vi "st_Poisson CDF (kx).vi"(10 "a":dbl=1.0, 11 "x":dbl=1.0) -> (0 "error":i32, 3 "cdf(x)":dbl=0.7357588823428847)   [LabVIEW 2020, in "NI_Gmath.lvlib"]
uses:
  <vilib>/gmath/NI_Gmath.lvlib
  <vilib>/gmath/statdist.llb/st_error_code.ctl
panel:
  # "Poisson CDF"
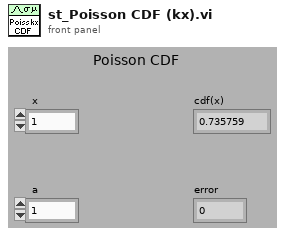
[diagram p1: front panel]
types:
  T1 = typedef "NI_Gmath.lvlib/st_error_code.ctl" = i32
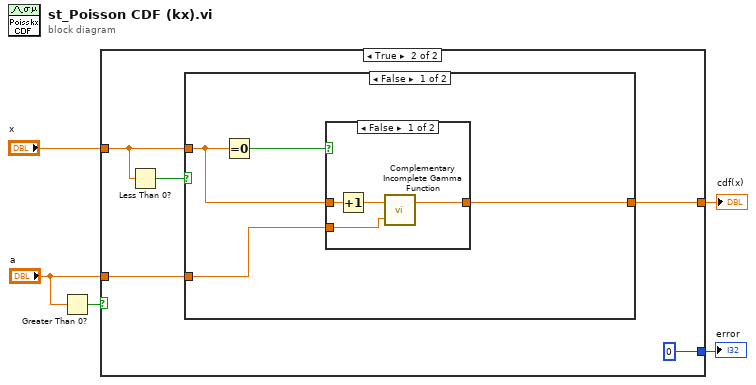
[diagram p0: block diagram]
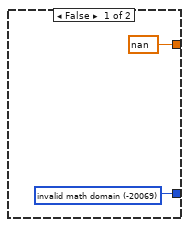
[diagram p2: hidden frame]
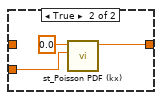
[diagram p3: hidden frame]
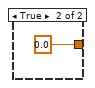
[diagram p4: hidden frame]
diagram:
  n1 = Greater Than 0?(x="a") -> (x > 0?=w1:bool)
  n2 = case shown="True" w1 {
    tunnel: [w6 0 ("invalid math domain")] -> w5
    tunnel: [nan w8] -> w4
    tunnel: "x" -> [_ w9]
    tunnel: "a" -> [_ w10]
    frame False {
      w6 = T1 -20069 items=["invalid math domain"=-20069, "Fourier interpolation size m >= n"=-20070, "empty array"=-20003] ("stat interp error code")
    }
    frame True {
      n3 = Less Than 0?(x=w9) -> (x < 0?=w11:bool)
      n4 = case shown="False" w11 {
        tunnel: [w13 0.0] -> w8
        tunnel: w10 -> [w14 _]
        tunnel: w9 -> [w16 _]
        frame False {
          n5 = Equal To 0?(x=w16) -> (x = 0?=w15:bool)
          n6 = case shown="False" w15 {
            tunnel: w16 -> [w20 _]
            tunnel: [w18 w21] -> w13
            tunnel: w14 -> [w17 w22]
            frame False {
              n7 = Increment(x=w20) -> (x+1=w19:dbl)
              n8 = call <vilib>:"Complementary Incomplete Gamma Function.vi"("a"=w17, "x"=w19) -> ("1 - g(x, a)"=w18:dbl)  [unwired: 1 in]
            }
            frame True {
              n9 = call <vilib>:"st_Poisson PDF (kx).vi"("a"=w22, "x"=0.0) -> ("pdf(x)"=w21:dbl)  [unwired: 8 in, 1 out]
            }
          }
        }
        frame True {
        }
      }
    }
  }
  "cdf(x)" <- w4
  "error" <- w5
